vi "Query Data as API String Arguments(variant).vi"(8 "error in":errorcluster, 9 "Setting Name":string, 11 "Internal Data":variant) -> (0 "error":errorcluster, 1 "Setting as String":string)   [LabVIEW 2017, in "API String Arguments Support.lvlib"]
uses:
  API String Arguments Support.lvlib
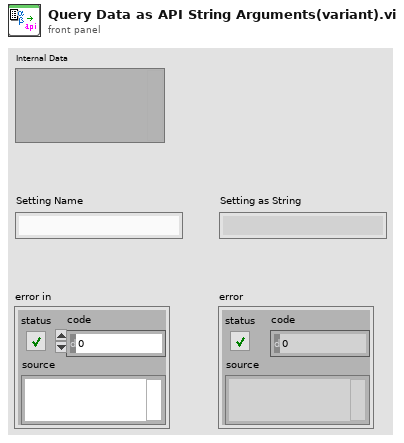
[diagram p1: front panel]
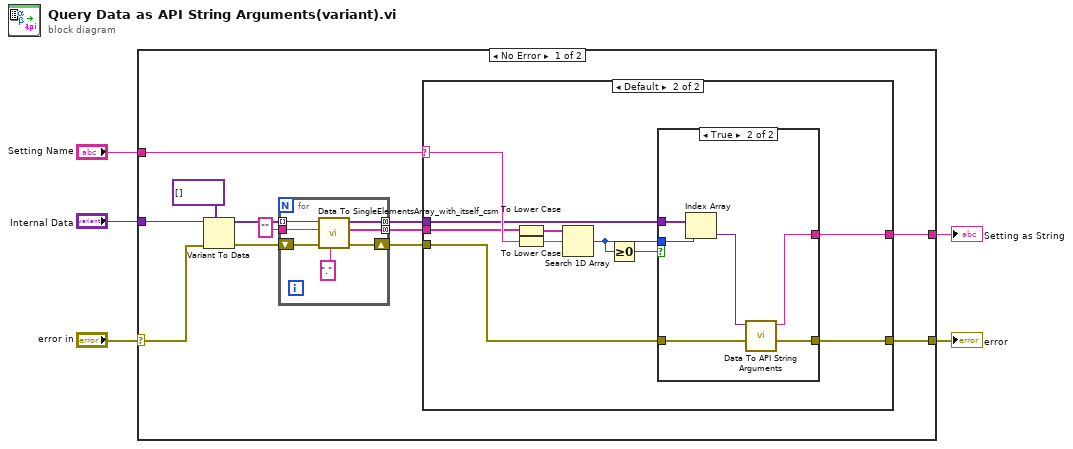
[diagram p0: block diagram]
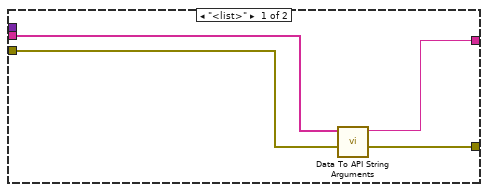
[diagram p2: hidden frame]
diagram:
  n1 = case shown="No Error" "error in" {
    selector: "error in" -> [w6 w46]
    tunnel: "Setting Name" -> [w17 _]
    tunnel: [w16 w46] -> w4
    tunnel: [w15 _] -> w3
    tunnel: "Internal Data" -> [w9 _]
    frame No Error {
      n2 = Variant To Data(error in=w6, type=variant[] [] ("Array"), Variant=w9) -> (data=w8:variant[], error out=w7:errorcluster)
      n3 = for {
        tunnel: [w43] -> w12 mode=concatenating
        tunnel: [w41] -> w13 mode=concatenating
        tunnel: "" ("parentUrl") -> [w40]
        tunnel: w8 -> [w39] mode=indexing
        shift-right: [w42] -> w11
        shift-left: w7 -> [w45]
        n4 = call "Data To SingleElementsArray_with_itself_csm.vi"("Seperator(/)"=".", "error in (no error)"=w45, "parentUrl"=w40, "Cluster"=w39) -> ("error out"=w42:errorcluster, "Full NameList"=w41:string[], "DataElementArray"=w43:variant[])  [unwired: 5 in]
      }
      n5 = case shown="Default" w17 {
        selector: w17 -> [_ w31]
        tunnel: [w18 w28] -> w16
        tunnel: [w21 w27] -> w15
        tunnel: w13 -> [w20 w24]
        tunnel: w12 -> [_ w23]
        tunnel: w11 -> [w19 w22]
        frame "<list>" {
          n6 = call "Data To API String Arguments.vi"("error in (no error)"=w19, "data"=w20) -> ("error out"=w18:errorcluster, "String"=w21:string)  [unwired: 8 in]
        }
        frame Default {
          n7 = To Lower Case(string=w24) -> (all lower case string=w30:string[])
          n8 = To Lower Case(string=w31) -> (all lower case string=w29:string)
          n9 = Search 1D Array(1D array=w30, element=w29) -> (index of element=w25:i32)  [unwired: 1 in]
          n10 = Greater Or Equal To 0?(x=w25) -> (x >= 0?=w26:bool)
          n11 = case shown="True" w26 {
            tunnel: w23 -> [_ w38]
            tunnel: w25 -> [_ w37]
            tunnel: w22 -> [w32 w35]
            tunnel: [w32 w33] -> w28
            tunnel: [_ w34] -> w27
            frame False {
            }
            frame True {
              n12 = Index Array(array=w38, index=w37) -> (element=w36:variant)
              n13 = call "Data To API String Arguments.vi"("error in (no error)"=w35, "data"=w36) -> ("error out"=w33:errorcluster, "String"=w34:string)  [unwired: 8 in]
            }
          }
        }
      }
    }
    frame Error {
    }
  }
  "Setting as String" <- w3
  "error" <- w4
